vi "PKG_IMC_HomeORG.vi"(0 "Handle":u32, 1 "riseEdge":i32, 2 "reducer":i32, 3 "hightvel":dbl, 5 "orgSW":i32, 7 "dir":i32, 8 "axis":i32, 9 "stopmode":i32, 10 "wait":i32, 12 "edir":i32, 13 "pos":i32, 14 "lowvel":dbl) -> (4 "Handle out":u32, 6 "function return":i32)   [LabVIEW 2011, in "IMC_Pkg4xxx.lvlib"]
doc: "PKG_IMC_HomeORG (IMC_HANDLE Handle, int orgSW, int dir, int stopmode, int riseEdge, int edir, int reducer, long pos, double hightvel, double lowvel, int wait, int axis);"
uses:
  IMC_Pkg4xxx.lvlib
  IMC_Pkg4xxx.dll
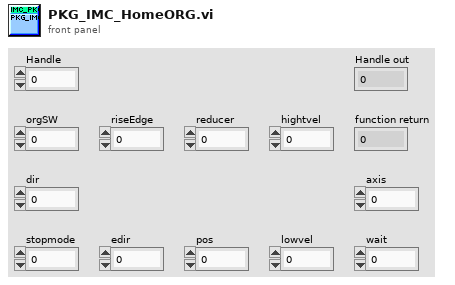
[diagram p1: front panel]
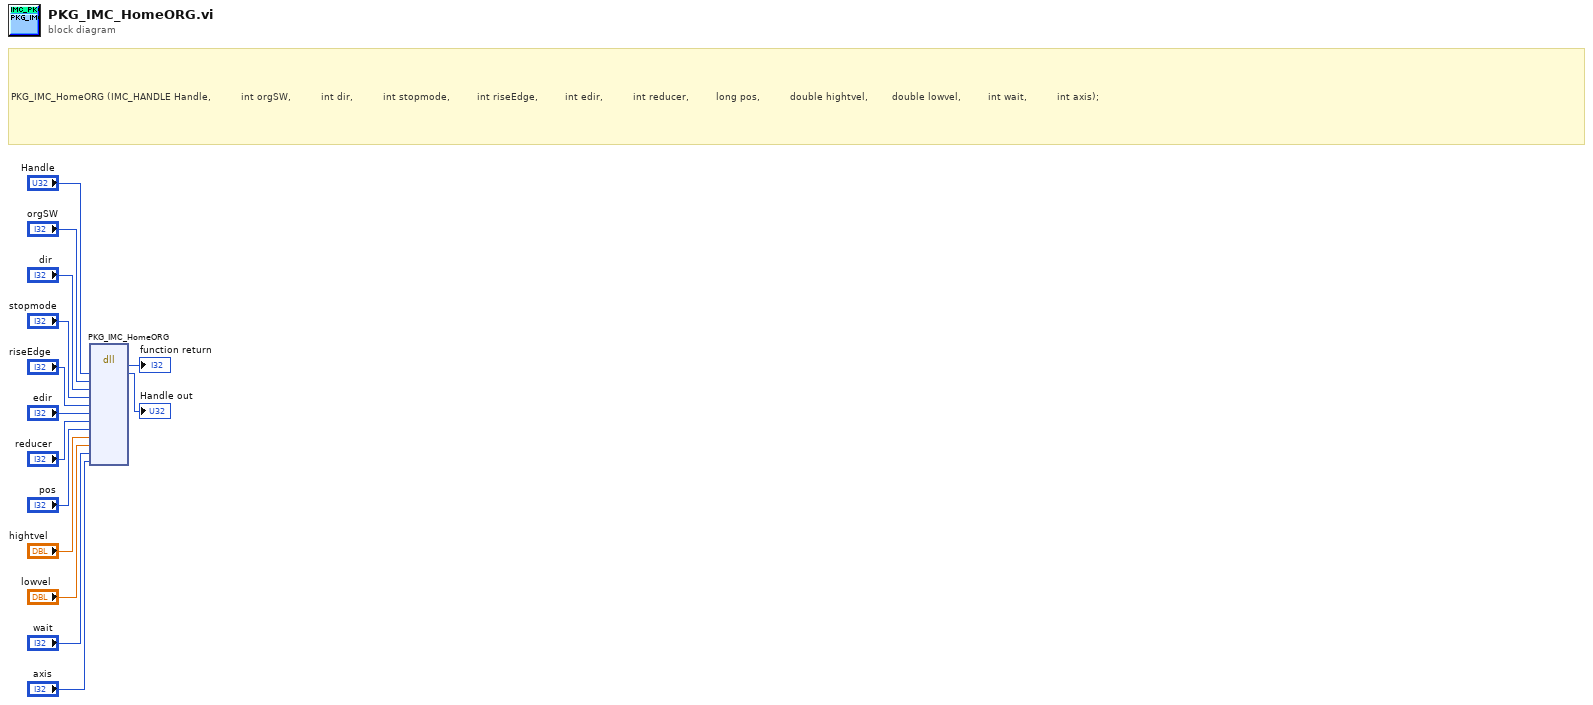
[diagram p0: block diagram]
diagram:
  # "PKG_IMC_HomeORG (IMC_HANDLE Handle,   \t\t\t\t\t\t\tint orgSW,\t\t\t\t\t\t\t\t\t\tint dir,\t\t\t\t\t\t\t\t\t\tint stopmode,\t\t\t\t\t\t\t\t\tint riseEdge,\t\t\t\t\t\t\t\t\tint edir,\t\t\t\t\t\t\t\t\t\tint reducer,\t\t\t\t\t\t\t\t\tlong pos,\t\t\t\t\t\t\t\t\t\tdouble hightvel,\t\t\t\t\t\t\t\tdouble lowvel,\t\t\t\t\t\t\t\t\tint wait,\t\t\t\t\t\t\t\t\t\tint axis);"
  n1 = dll-call lib="PTH1mabs F光盘刻录\niMC MotionIMCNet_V4.0IMCAppincLabviewIMC_PKG4xxxIMC_PKG4xxx\nIMC_Pkg4xxx.*" fn="PKG_IMC_HomeORG"("Handle"="Handle", "orgSW"="orgSW", "dir"="dir", "stopmode"="stopmode", "riseEdge"="riseEdge", "edir"="edir", "reducer"="reducer", "pos"="pos", "hightvel"="hightvel", "lowvel"="lowvel", "wait"="wait", "axis"="axis") -> (→"function return":i32, "Handle"=→"Handle out":u32)  [unwired: 14 in, 2 out]
